vi "UpdateSomeMenuBarContent.vi"(8 "error in (no error)":errorcluster, 10 "menu ref":refnum<k9>, 11 "Gviewer in":refnum<class "Gviewer.lvclass">) -> (0 "error out":errorcluster, 3 "Gviewer out":refnum<class "Gviewer.lvclass">)   [LabVIEW 2020, in "Sgraph_lib_V1.lvlib" / "Gviewer.lvclass"]
uses:
  Gviewer.lvclass
  Gviewer.lvclass/Gviewer.ctl
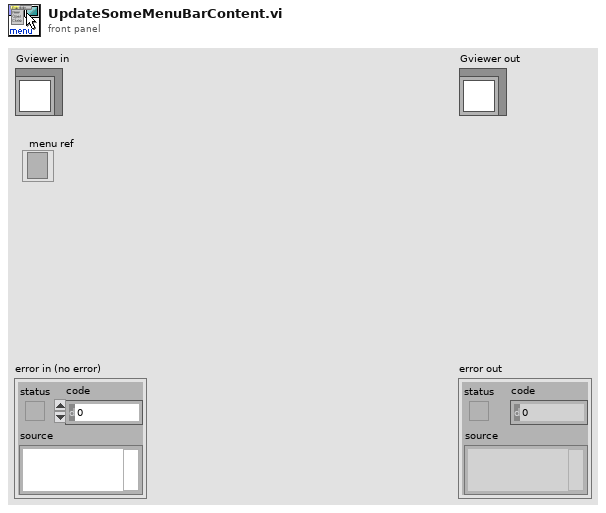
[diagram p1: front panel]
types:
  T1 = typedef "MenuItem.ctl" = cluster{"name":string, "tag":string, "checked":bool, "enabled":bool}
  T2 = typedef "MenuStructure.ctl" = cluster{"After_tag":string, "MenuItems":T1[]}[]
  T3 = typedef "Sgraph_lib_V1.lvlib/Gviewer.lvclass/MinMax.ctl" = enum16{"On", "Off", "Focus"}
  T4 = typedef "Sgraph_lib_V1.lvlib/Gviewer.lvclass/TD_Lscale.ctl" = enum16{"none", "one", "many"}
  T5 = typedef "Sgraph_lib_V1.lvlib/Gviewer.lvclass/TD_Rscale.ctl" = enum16{"none", "one", "all"}
  T6 = typedef "Sgraph_lib_V1.lvlib/Gviewer.lvclass/YgraphDef.ctl" = cluster{"Plot":i32, "X(%)":dbl}
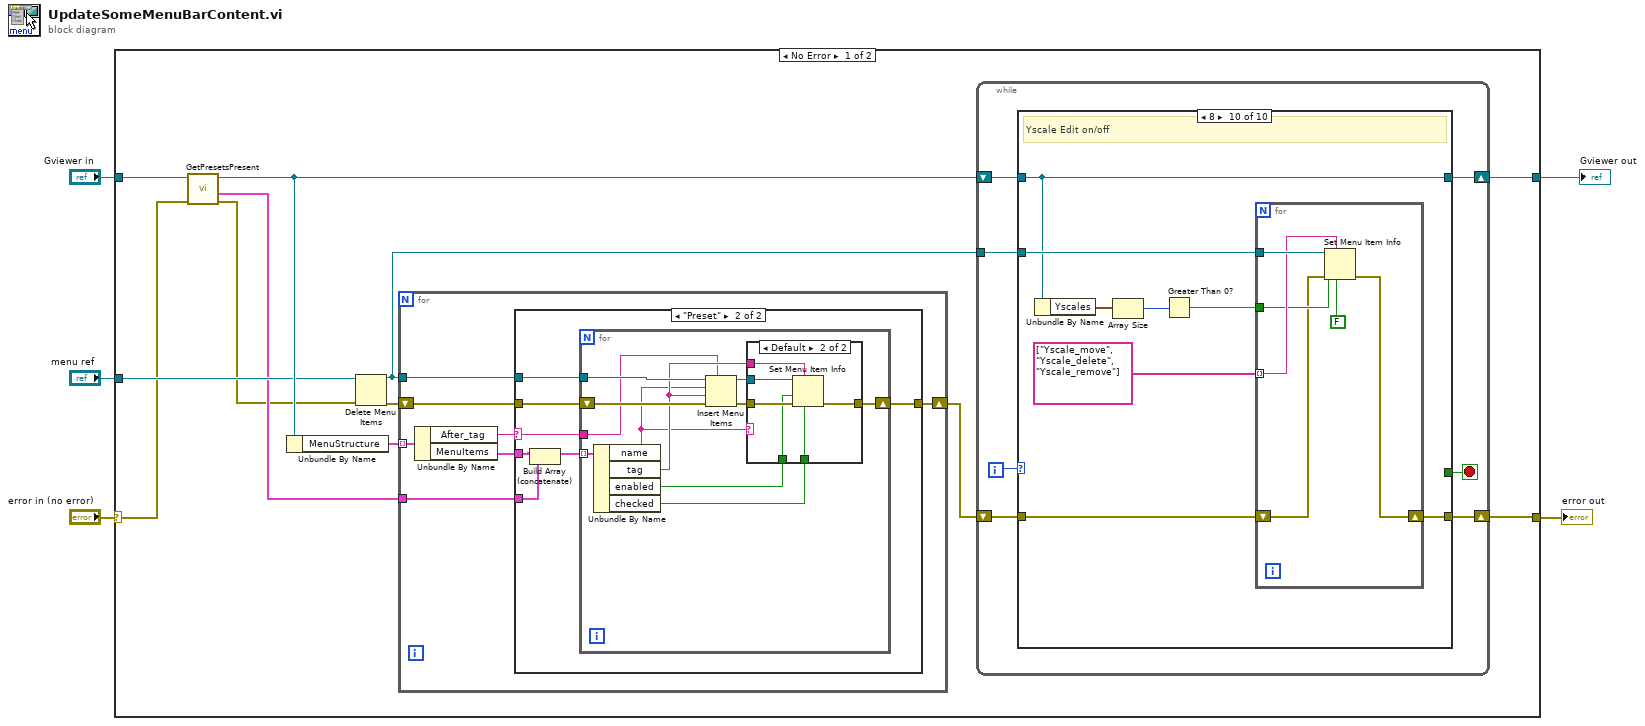
[diagram p0: block diagram]
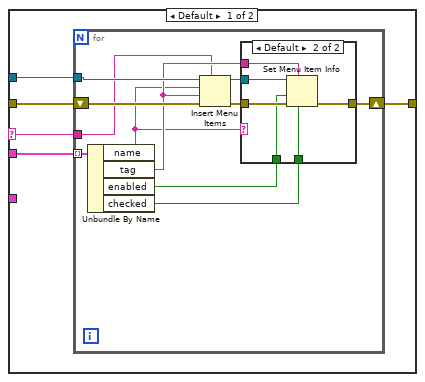
[diagram p2: hidden frame]
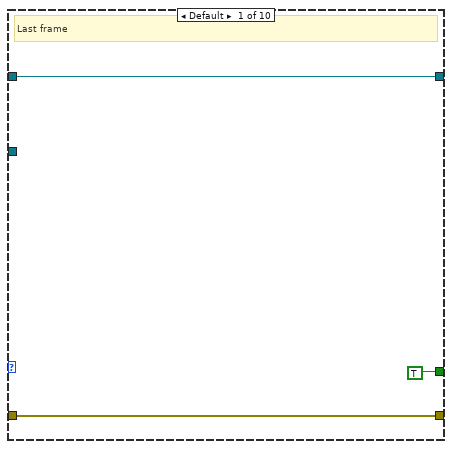
[diagram p5: hidden frame]
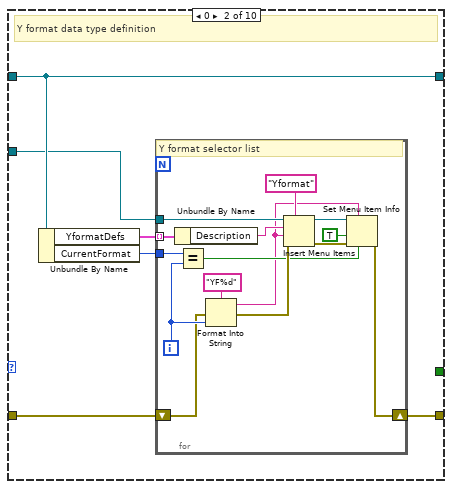
[diagram p6: hidden frame]
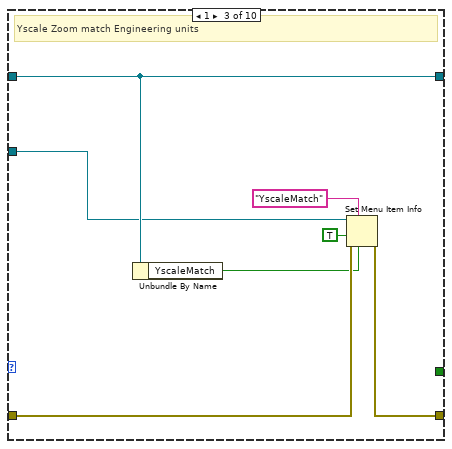
[diagram p7: hidden frame]
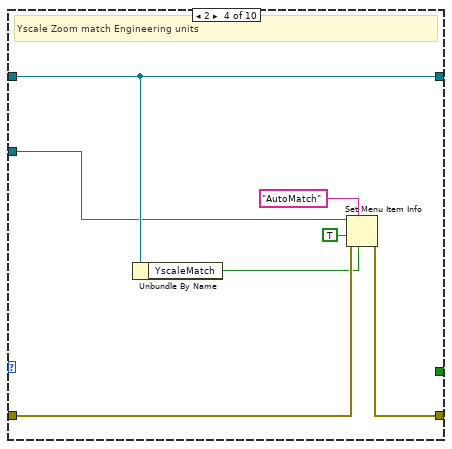
[diagram p8: hidden frame]
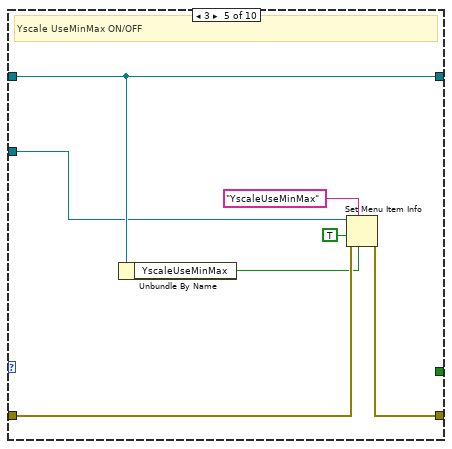
[diagram p9: hidden frame]
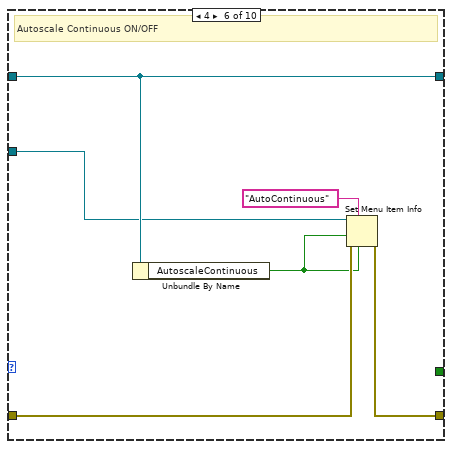
[diagram p10: hidden frame]
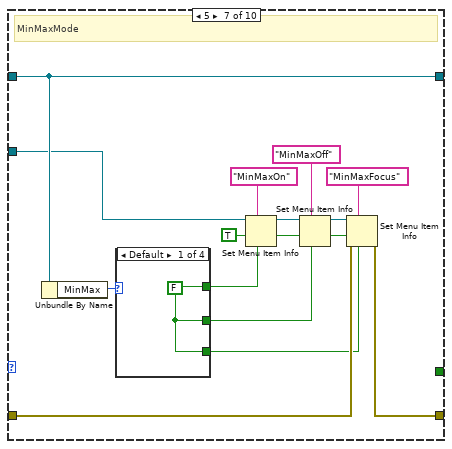
[diagram p11: hidden frame]
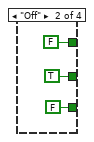
[diagram p12: hidden frame]
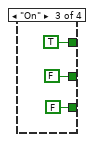
[diagram p13: hidden frame]
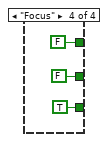
[diagram p14: hidden frame]
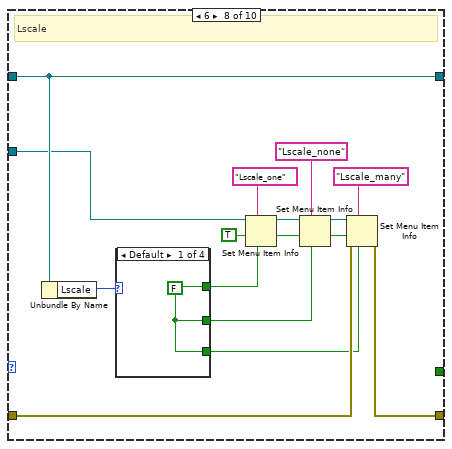
[diagram p15: hidden frame]
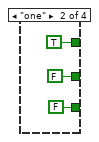
[diagram p16: hidden frame]
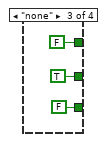
[diagram p17: hidden frame]
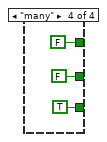
[diagram p18: hidden frame]
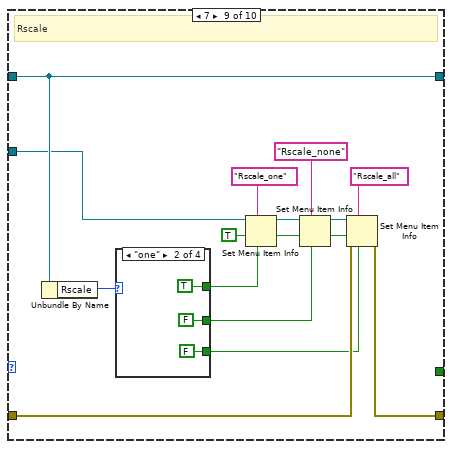
[diagram p19: hidden frame]
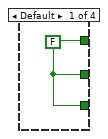
[diagram p20: hidden frame]
diagram:
  n1 = case shown="No Error" "error in (no error)" {
    selector: "error in (no error)" -> [w10 w217]
    tunnel: [w14 w217] -> w4
    tunnel: [w15 w216] -> w2
    tunnel: "Gviewer in" -> [w12 w216]
    tunnel: "menu ref" -> [w13 _]
    frame No Error {
      n2 = call "GetPresetsPresent.vi"("error in (no error)"=w10, "Gviewer in"=w12) -> ("error out"=w9:errorcluster, "PresentsInMenu"=w11:T1[], "Gviewer out"=w15:refnum<class "Gviewer.lvclass">)  [unwired: 7 in]
      n3 = Unbundle By Name(w15) -> ("MenuStructure"=w8:T2)
      n4 = Delete Menu Items(6:w9, 9:w13) -> (0:w7:errorcluster, 3:w6:refnum<k9>)  [unwired: 2 in]
      n5 = for {
        tunnel: w8 -> [w23] mode=indexing
        shift-right: [w19] -> w16
        shift-left: w7 -> [w20]
        tunnel: w6 -> [w18]
        tunnel: w11 -> [w17]
        n6 = Unbundle By Name(w23) -> ("After_tag"=w21:string, "MenuItems"=w22:T1[])
        n7 = case shown="\"Preset\"" w21 {
          selector: w21 -> [w27 w53]
          tunnel: w22 -> [w28 w48]
          tunnel: w20 -> [w26 w52]
          tunnel: [w25 w51] -> w19
          tunnel: w18 -> [w24 w50]
          tunnel: w17 -> [_ w49]
          frame Default {
            n8 = for {
              tunnel: w28 -> [w36] mode=indexing
              tunnel: w27 -> [w30]
              shift-right: [w37] -> w25
              shift-left: w26 -> [w39]
              tunnel: w24 -> [w35]
              n9 = Unbundle By Name(w36) -> ("name"=w29:string, "tag"=w31:string, "enabled"=w32:bool, "checked"=w33:bool)
              n10 = Insert Menu Items(5:w30, 6:w39, 7:w31, 8:w29, 9:w35) -> (0:w38:errorcluster, 3:w34:refnum<k9>)  [unwired: 1 in, 1 out]
              n11 = case shown="Default" w29 {
                tunnel: w38 -> [w40 w46]
                tunnel: [w40 w45] -> w37
                tunnel: w34 -> [_ w44]
                tunnel: w33 -> [_ w43]
                tunnel: w32 -> [_ w42]
                tunnel: w31 -> [_ w41]
                frame "app_separator" {
                }
                frame Default {
                  n12 = Set Menu Item Info(6:w43, 7:w41, 8:w46, 9:w42, 11:w44) -> (0:w45:errorcluster)  [unwired: 2 in, 1 out]
                }
              }
            }
          }
          frame "Preset" {
            n13 = Build Array (concatenate)(w48, w49) -> (w47:T1[])
            n14 = for {
              tunnel: w47 -> [w61] mode=indexing
              tunnel: w53 -> [w55]
              shift-right: [w62] -> w51
              shift-left: w52 -> [w64]
              tunnel: w50 -> [w60]
              n15 = Unbundle By Name(w61) -> ("name"=w54:string, "tag"=w56:string, "enabled"=w57:bool, "checked"=w58:bool)
              n16 = Insert Menu Items(5:w55, 6:w64, 7:w56, 8:w54, 9:w60) -> (0:w63:errorcluster, 3:w59:refnum<k9>)  [unwired: 1 in, 1 out]
              n17 = case shown="Default" w54 {
                tunnel: w63 -> [w65 w71]
                tunnel: [w65 w70] -> w62
                tunnel: w59 -> [_ w69]
                tunnel: w58 -> [_ w68]
                tunnel: w57 -> [_ w67]
                tunnel: w56 -> [_ w66]
                frame "app_separator" {
                }
                frame Default {
                  n18 = Set Menu Item Info(6:w68, 7:w66, 8:w71, 9:w67, 11:w69) -> (0:w70:errorcluster)  [unwired: 2 in, 1 out]
                }
              }
            }
          }
        }
      }
      n19 = while {
        shift-right: [w77] -> w14
        shift-left: w16 -> [w78]
        shift-right: [w74] -> _
        shift-left: w15 -> [w76]
        tunnel: w6 -> [w72]
        i -> [w75]
        stop <- w73 stop-if-true
        n20 = case shown="8" w75 {
          tunnel: w78 -> [w80 w87 w107 w114 w121 w128 w142 w166 w190 w205]
          tunnel: [w80 w86 w109 w116 w123 w129 w143 w167 w191 w204] -> w77
          tunnel: w76 -> [w81 w83 w105 w112 w119 w126 w140 w164 w188 w202]
          tunnel: [w81 w83 w105 w112 w119 w126 w140 w164 w188 w202] -> w74
          tunnel: [TRUE _ _ _ _ _ _ _ _ _] -> w73
          tunnel: w72 -> [_ w82 w103 w110 w117 w124 w130 w154 w178 w203]
          frame Default {
            # "Last frame"
          }
          frame 0 {
            # "Y format data type definition"
            n21 = Unbundle By Name(w83) -> ("YformatDefs"=w85:cluster{"Description":string, "Format":string}[], "CurrentFormat"=w84:i32)
            n22 = for {
              shift-right: [w88] -> w86
              shift-left: w87 -> [w95]
              tunnel: w85 -> [w101] mode=indexing
              tunnel: w84 -> [w102]
              tunnel: w82 -> [w100]
              i -> [w97]
              # "Y format selector list"
              n23 = Unbundle By Name(w101) -> ("Description"=w98:string)
              n24 = Equal?(x=w102, y=w97) -> (x = y?=w91:bool)
              n25 = Format Into String(format string="YF%d", error in=w95, w97) -> (resulting string=w90:string, error out=w94:errorcluster)  [unwired: 1 in]
              n26 = Insert Menu Items(5:"Yformat" ("menu tag"), 6:w94, 7:w90, 8:w98, 9:w100) -> (0:w93:errorcluster, 3:w89:refnum<k9>)  [unwired: 1 in, 1 out]
              n27 = Set Menu Item Info(6:w91, 7:w90, 8:w93, 9:TRUE ("enabled"), 11:w89) -> (0:w88:errorcluster)  [unwired: 2 in, 1 out]
            }
          }
          frame 1 {
            # "Yscale Zoom match Engineering units"
            n28 = Unbundle By Name(w105) -> ("YscaleMatch"=w104:bool)
            n29 = Set Menu Item Info(6:w104, 7:"YscaleMatch" ("menu tag"), 8:w107, 9:TRUE ("enabled"), 11:w103) -> (0:w109:errorcluster)  [unwired: 2 in, 1 out]
          }
          frame 2 {
            # "Yscale Zoom match Engineering units"
            n30 = Unbundle By Name(w112) -> ("YscaleMatch"=w111:bool)
            n31 = Set Menu Item Info(6:w111, 7:"AutoMatch" ("menu tag"), 8:w114, 9:TRUE ("enabled"), 11:w110) -> (0:w116:errorcluster)  [unwired: 2 in, 1 out]
          }
          frame 3 {
            # "Yscale UseMinMax ON/OFF"
            n32 = Unbundle By Name(w119) -> ("YscaleUseMinMax"=w118:bool)
            n33 = Set Menu Item Info(6:w118, 7:"YscaleUseMinMax" ("menu tag"), 8:w121, 9:TRUE ("enabled"), 11:w117) -> (0:w123:errorcluster)  [unwired: 2 in, 1 out]
          }
          frame 4 {
            # "Autoscale Continuous ON/OFF"
            n34 = Unbundle By Name(w126) -> ("AutoscaleContinuous"=w125:bool)
            n35 = Set Menu Item Info(6:w125, 7:"AutoContinuous" ("menu tag"), 8:w128, 9:w125, 11:w124) -> (0:w129:errorcluster)  [unwired: 2 in, 1 out]
          }
          frame 5 {
            w135 = TRUE ("enabled")
            # "MinMaxMode"
            n36 = Unbundle By Name(w140) -> ("MinMax"=w134:T3)
            n37 = case shown="Default" w134 {
              tunnel: [w144 FALSE ("enabled") TRUE ("enabled") FALSE ("enabled")] -> w133
              tunnel: [w144 TRUE ("enabled") FALSE ("enabled") FALSE ("enabled")] -> w132
              tunnel: [w144 FALSE ("enabled") FALSE ("enabled") TRUE ("enabled")] -> w131
              frame Default {
                w144 = FALSE ("enabled")
              }
              frame "Off" {
              }
              frame "On" {
              }
              frame "Focus" {
              }
            }
            n38 = Set Menu Item Info(6:w133, 7:"MinMaxOn" ("menu tag"), 9:w135, 11:w130) -> (3:w139:refnum<k9>)  [unwired: 3 in, 1 out]
            n39 = Set Menu Item Info(6:w132, 7:"MinMaxOff" ("menu tag"), 9:w135, 11:w139) -> (3:w138:refnum<k9>)  [unwired: 3 in, 1 out]
            n40 = Set Menu Item Info(6:w131, 7:"MinMaxFocus" ("menu tag"), 8:w142, 9:w135, 11:w138) -> (0:w143:errorcluster)  [unwired: 2 in, 1 out]
          }
          frame 6 {
            w159 = TRUE ("enabled")
            # "Lscale"
            n41 = Unbundle By Name(w164) -> ("Lscale"=w158:T4)
            n42 = case shown="Default" w158 {
              tunnel: [w168 TRUE ("enabled") FALSE ("enabled") FALSE ("enabled")] -> w157
              tunnel: [w168 FALSE ("enabled") TRUE ("enabled") FALSE ("enabled")] -> w156
              tunnel: [w168 FALSE ("enabled") FALSE ("enabled") TRUE ("enabled")] -> w155
              frame Default {
                w168 = FALSE ("enabled")
              }
              frame "one" {
              }
              frame "none" {
              }
              frame "many" {
              }
            }
            n43 = Set Menu Item Info(6:w157, 7:"Lscale_one" ("menu tag"), 9:w159, 11:w154) -> (3:w163:refnum<k9>)  [unwired: 3 in, 1 out]
            n44 = Set Menu Item Info(6:w156, 7:"Lscale_none" ("menu tag"), 9:w159, 11:w163) -> (3:w162:refnum<k9>)  [unwired: 3 in, 1 out]
            n45 = Set Menu Item Info(6:w155, 7:"Lscale_many" ("menu tag"), 8:w166, 9:w159, 11:w162) -> (0:w167:errorcluster)  [unwired: 2 in, 1 out]
          }
          frame 7 {
            w183 = TRUE ("enabled")
            # "Rscale"
            n46 = Unbundle By Name(w188) -> ("Rscale"=w182:T5)
            n47 = case shown="\"one\"" w182 {
              tunnel: [w192 TRUE ("enabled") FALSE ("enabled") FALSE ("enabled")] -> w181
              tunnel: [w192 FALSE ("enabled") TRUE ("enabled") FALSE ("enabled")] -> w180
              tunnel: [w192 FALSE ("enabled") FALSE ("enabled") TRUE ("enabled")] -> w179
              frame Default {
                w192 = FALSE ("enabled")
              }
              frame "one" {
              }
              frame "none" {
              }
              frame "all" {
              }
            }
            n48 = Set Menu Item Info(6:w181, 7:"Rscale_one" ("menu tag"), 9:w183, 11:w178) -> (3:w187:refnum<k9>)  [unwired: 3 in, 1 out]
            n49 = Set Menu Item Info(6:w180, 7:"Rscale_none" ("menu tag"), 9:w183, 11:w187) -> (3:w186:refnum<k9>)  [unwired: 3 in, 1 out]
            n50 = Set Menu Item Info(6:w179, 7:"Rscale_all" ("menu tag"), 8:w190, 9:w183, 11:w186) -> (0:w191:errorcluster)  [unwired: 2 in, 1 out]
          }
          frame 8 {
            # "Yscale Edit on/off"
            n51 = Unbundle By Name(w202) -> ("Yscales"=w207:T6[])
            n52 = Array Size(array=w207) -> (size(s)=w208:i32)
            n53 = Greater Than 0?(x=w208) -> (x > 0?=w209:bool)
            n54 = for {
              tunnel: string[] ["Yscale_move", "Yscale_delete", "Yscale_remove"] -> [w214] mode=indexing
              tunnel: w203 -> [w215]
              tunnel: w209 -> [w212]
              shift-right: [w210] -> w204
              shift-left: w205 -> [w211]
              n55 = Set Menu Item Info(6:FALSE ("checked"), 7:w214, 8:w211, 9:w212, 11:w215) -> (0:w210:errorcluster)  [unwired: 2 in, 1 out]
            }
          }
        }
      }
    }
    frame Error {
    }
  }
  "error out" <- w4
  "Gviewer out" <- w2
